vi "Special 2 Step 4 (SubVI).vi"(0 "Rdist":dbl, 5 "rblc":dbl, 7 "aRB":dbl, 9 "aRB1":dbl, 11 "aRB2":dbl) -> (4 "lcx2":dbl, 6 "lcy2":dbl, 8 "rcx2":dbl, 10 "rcy2":dbl, 15 "aRB1+aRB2":dbl)   [LabVIEW 2015]
uses:
  <vilib>/express/express arith-compare/Formula/XNode/ExpressFormulaBlockNode.xnode
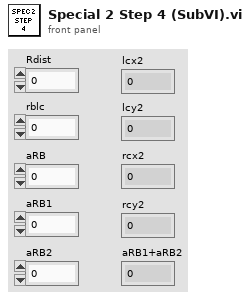
[diagram p1: front panel]
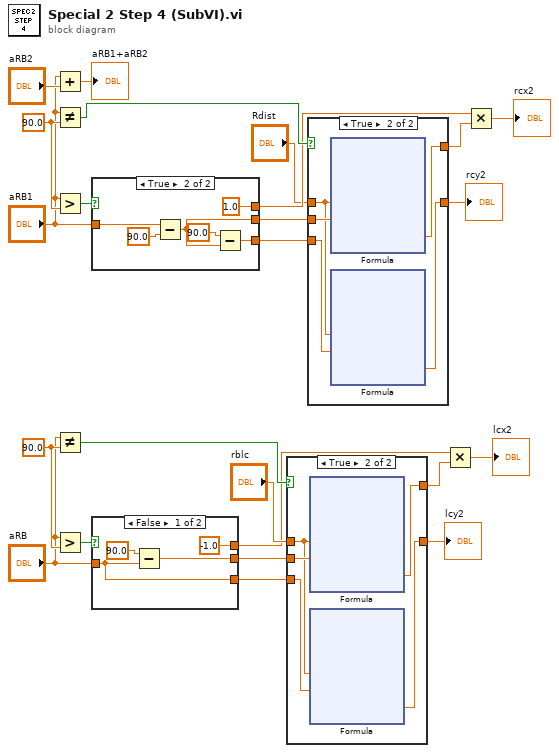
[diagram p0: block diagram]
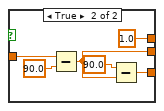
[diagram p2: hidden frame]
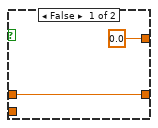
[diagram p3: hidden frame]
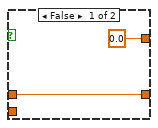
[diagram p4: hidden frame]
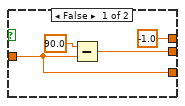
[diagram p5: hidden frame]
diagram:
  w18 = 90.0 ("y")
  w19 = 90.0 ("y")
  n1 = Add(x="aRB1", y="aRB2") -> (x+y=→"aRB1+aRB2":dbl)
  n2 = Not Equal?(x="aRB1", y=w19) -> (x != y?=w21:bool)
  n3 = Greater?(x="aRB1", y=w19) -> (0:w22:bool)
  n4 = Not Equal?(x="aRB", y=w18) -> (x != y?=w20:bool)
  n5 = Greater?(x="aRB", y=w18) -> (0:w7:bool)
  n6 = case shown="True" w22 {
    tunnel: "aRB1" -> [w26 w34]
    tunnel: [w27 w31] -> w16
    tunnel: [w26 w30] -> w17
    tunnel: [-1.0 1.0] -> w12
    frame False {
      n7 = Subtract(x=90.0, y=w26) -> (x-y=w27:dbl)
    }
    frame True {
      n8 = Subtract(x=w34, y=90.0) -> (x-y=w31:dbl)
      n9 = Subtract(x=90.0, y=w31) -> (x-y=w30:dbl)
    }
  }
  n10 = case shown="False" w7 {
    tunnel: "aRB" -> [w36 w44]
    tunnel: [w37 w41] -> w14
    tunnel: [w36 w40] -> w15
    tunnel: [-1.0 1.0] -> w9
    frame False {
      n11 = Subtract(x=90.0, y=w36) -> (x-y=w37:dbl)
    }
    frame True {
      n12 = Subtract(x=w44, y=90.0) -> (x-y=w41:dbl)
      n13 = Subtract(x=90.0, y=w41) -> (x-y=w40:dbl)
    }
  }
  n14 = case shown="True" w20 {
    tunnel: w15 -> [_ w51]
    tunnel: w14 -> [_ w50]
    tunnel: [0.0 ("Result") w49] -> w8
    tunnel: [w46 w48] -> w4
    tunnel: "rblc" -> [w46 w47]
    frame False {
    }
    frame True {
      n15 = xnode "Formula"("rblc"=w47, "aLX"=w50) -> ("Result"=w49:dbl)  [unwired: 1 in, 1 out]
      n16 = xnode "Formula"("rblc"=w47, "aLY"=w51) -> ("Result"=w48:dbl)  [unwired: 1 in, 1 out]
    }
  }
  "lcy2" <- w4
  n17 = case shown="True" w21 {
    tunnel: w17 -> [_ w78]
    tunnel: w16 -> [_ w77]
    tunnel: [0.0 ("Result") w76] -> w13
    tunnel: [w73 w75] -> w3
    tunnel: "Rdist" -> [w73 w74]
    frame False {
    }
    frame True {
      n18 = xnode "Formula"("Rdist"=w74, "aRX"=w77) -> ("Result"=w76:dbl)  [unwired: 1 in, 1 out]
      n19 = xnode "Formula"("Rdist"=w74, "aRY"=w78) -> ("Result"=w75:dbl)  [unwired: 1 in, 1 out]
    }
  }
  "rcy2" <- w3
  n20 = Multiply(x=w9, y=w8) -> (x*y=→"lcx2":dbl)
  n21 = Multiply(x=w12, y=w13) -> (x*y=→"rcx2":dbl)
